vi "Reset Timeout.vi"(8 "error in (no error)":errorcluster, 11 "Automation Controller in":refnum<class "Automation Controller.lvclass">) -> (0 "error out":errorcluster, 3 "State Machine Actor out":refnum<class "State Machine Actor.lvclass">)   [LabVIEW 2024, in "Automation Controller.lvlib" / "Automation Controller.lvclass"]
uses:
  Automation Controller.lvclass
  Automation Controller.lvclass/Automation Controller.ctl
  Timed Out/Timed Out/Timed Out.lvclass
  Idle/Idle/Idle.lvclass
  C:/Users/uspoaotto/OneDrive - Oregon Tool/Desktop/working copies/stateMachineActor/src/State Machine Actor/State Machine Actor/State Machine Actor.lvclass
  C:/Users/uspoaotto/OneDrive - Oregon Tool/Desktop/working copies/stateMachineActor/src/_State Machine Actor/_State Machine Actor/_State Machine Actor.lvclass
  C:/Program Files (x86)/National Instruments/LabVIEW 2024/vi.lib/ActorFramework/Actor/Actor.lvclass
  C:/Users/uspoaotto/OneDrive - Oregon Tool/Desktop/working copies/stateMachineActor/src/Automation Controller/Automation Controller/Automation Controller.lvclass
  State Machine Actor/State Machine Actor/State Machine Actor.lvclass
  C:/Users/uspoaotto/OneDrive - Oregon Tool/Desktop/working copies/stateMachineActor/src/Timed Out/Timed Out/Timed Out.lvclass
  C:/Users/uspoaotto/OneDrive - Oregon Tool/Desktop/working copies/stateMachineActor/src/Idle/Idle/Idle.lvclass
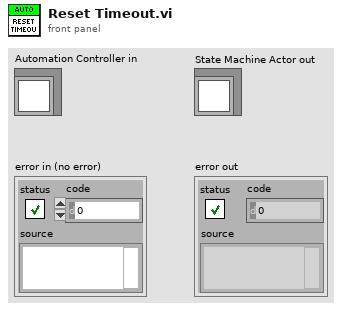
[diagram p1: front panel]
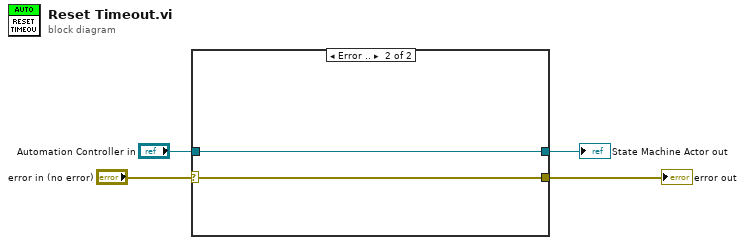
[diagram p0: block diagram]
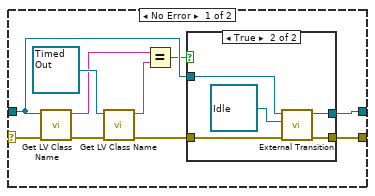
[diagram p2: hidden frame]
diagram:
  n1 = case shown="Error .." "error in (no error)" {
    selector: "error in (no error)" -> [w8 w22]
    tunnel: "Automation Controller in" -> [w11 w23]
    tunnel: [w10 w23] -> w2
    tunnel: [w6 w22] -> w1
    frame No Error {
      n2 = call <vilib>:"Get LV Class Name.vi"("error in (no error)"=w8, "object"=w11) -> ("error out"=w9:errorcluster, "class name"=w13:string)  [unwired: 8 in]
      n3 = call <vilib>:"Get LV Class Name.vi"("error in (no error)"=w9, "object"=refnum<class "Timed Out.lvclass"> refnum ("Timed Out.lvlib:Timed Out.lvclass")) -> ("error out"=w7:errorcluster, "class name"=w12:string)  [unwired: 8 in]
      n4 = Equal?(x=w13, y=w12) -> (x = y?=w5:bool)
      n5 = case shown="True" w5 {
        tunnel: w11 -> [w15 w21]
        tunnel: [w15 w20] -> w10
        tunnel: w7 -> [w16 w18]
        tunnel: [w16 w17] -> w6
        frame False {
        }
        frame True {
          n6 = call-dynamic "External Transition.vi"("error in (no error)"=w18, "Target State in"=refnum<class "Idle.lvclass"> refnum ("Idle.lvlib:Idle.lvclass"), "State Machine Actor in"=w21) -> ("error out"=w17:errorcluster, "State Machine Actor out"=w20:refnum<class "State Machine Actor.lvclass">)  [unwired: 7 in]
        }
      }
    }
    frame Error {
    }
  }
  "error out" <- w1
  "State Machine Actor out" <- w2
